vi "27_Reversal of no in array.vi"() -> ()   [LabVIEW 2018]
panel:
  out "Reversed Array":dbl[](array[numeric])
  out "Maximum":dbl
  out "Minimum":dbl
  out "Array":dbl[](array[numeric])
  # "WAP to generate 5 numbers. Reverse the array and then find the min and max of them"
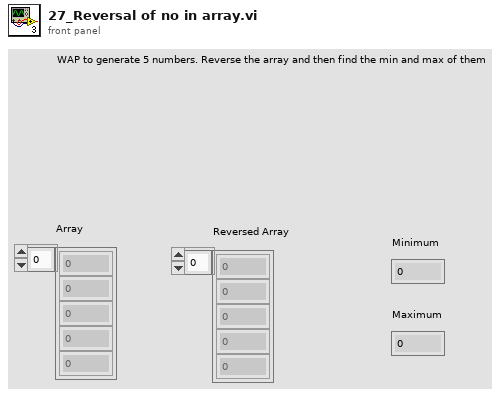
[diagram p1: front panel]
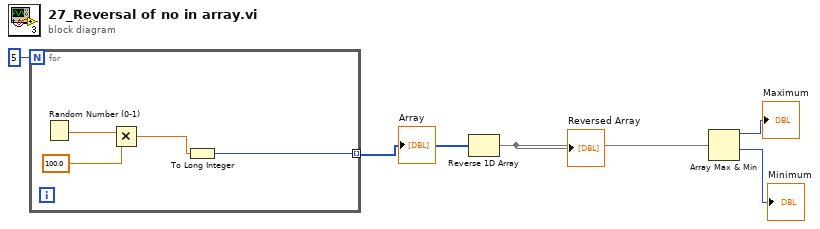
[diagram p0: block diagram]
diagram:
  n1 = for {
    N: 5 -> [_]
    tunnel: [w7] -> w2 mode=indexing
    n2 = Random Number (0-1)() -> (number: 0 to 1=w9:dbl)
    n3 = Multiply(x=w9, y=100.0 ("x")) -> (x*y=w8:dbl)
    n4 = To Long Integer(number=w8) -> (32bit integer=w7:i32)
  }
  "Array" <- w2
  n5 = Reverse 1D Array(array=w2) -> (reversed array=w1:i32[])
  "Reversed Array" <- w1
  n6 = Array Max & Min(array=w1) -> (max value=→"Maximum":i32, min value=→"Minimum":i32)  [unwired: 2 out]
